vi "General-PrintHistogram.vi"(1 "Image":T1) -> (0 "XY Graph":cluster{sgl[], "histogram":u32[]}(graph))   [LabVIEW 2010]
uses:
  <vilib>/vision/Image Controls.llb/IMAQ Image.ctl
  <vilib>/vision/NI_Vision_Development_Module.lvlib
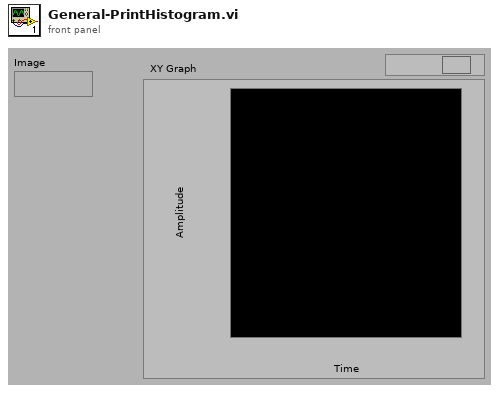
[diagram p1: front panel]
types:
  T1 = typedef "IMAQ Image.ctl" = refnum<image>
  T2 = cluster{"histogram":u32[], "Minimal Value":sgl, "Maximal Value":sgl, "Starting Value":sgl, "Interval Width":sgl, "Mean Value":sgl, "Standard  Variation":sgl, "Area (pixels)":i32}
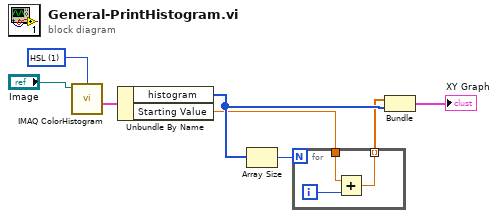
[diagram p0: block diagram]
diagram:
  w1 = u16 1 items=["RGB", "HSL", "HSV", "HSI"] ("Color Mode")
  n1 = call "IMAQ ColorHistogram"("Color Mode"=w1, "Image Src"="Image") -> ("Blue or Luma or Val or Inten or Z or b* Histogram Report"=w3:T2)  [unwired: 4 in, 3 out]
  n2 = Unbundle By Name(w3) -> ("histogram"=w8:u32[], "Starting Value"=w4:sgl)
  n3 = Array Size(array=w8) -> (size(s)=w5:i32)
  n4 = for {
    N: w5 -> [_]
    tunnel: w4 -> [w10]
    tunnel: [w9] -> w7 mode=indexing
    i -> [w11]
    n5 = Add(x=w10, y=w11) -> (x+y=w9:sgl)
  }
  n6 = Bundle(w7, "histogram"=w8) -> (→"XY Graph":cluster{sgl[], "histogram":u32[]})  [unwired: 1 in]
